vi "AMI_SetCampo.vi"(6 "error in (no error)":errorcluster, 7 "Index":i8) -> (0 "error out":errorcluster, 1 "resulting string Z":string="Set Magnetic Field 1000.000Tesla at 100.000Tesla/min, Linear, Persistent, Sweep&meas", 2 "resulting string Y":string="Set Magnetic Field 1000.000Tesla at 100.000Tesla/min, Linear, Persistent, Sweep&meas", 3 "resulting string X":string="Set Magnetic Field 1000.000Tesla at 100.000Tesla/min, Linear, Persistent, Sweep&meas")   [LabVIEW 2017]
doc: "Use this template to create a dialog box. This template polls the state of the buttons on the front panel and does not use events. Use the Dialog Using Events template (not available in Base package) to create a dialog box with event handling."
panel:
  out "Z Field Units":u16(ring)=1 items=["KGauss", "Tesla"]
  out "Z Ramp Units":u16(ring)=1 items=["Per SECOND", "Per MINUTE"]
  out "Y Field Units":u16(ring)=1 items=["KGauss", "Tesla"]
  out "Y Ramp Units":u16(ring)=1 items=["Per SECOND", "Per MINUTE"]
  in  "Z campo":dbl=0.1
  in  "Z rate":dbl=0.03
  in  "Y campo":dbl=0.1
  in  "Y rate":dbl=0.03
  in  "Modo Rampa":u16(ring)=1 items=["RAMP", "PAUSE", "MANUAL UP", "MANUAL DOWN", "ZERO"]
  out "X Ramp Units":u16(ring)=1 items=["Per SECOND", "Per MINUTE"]
  out "X Field Units":u16(ring)=1 items=["KGauss", "Tesla"]
  out "Wait stability":bool=TRUE
  in  "Field Mode":i32(ring) items=["Persistent", "Driven"]
  in  "Approach":i32(ring) items=["Linear", "NoOvershoot", "Oscillate"]
  in  "X rate":dbl=0.03
  in  "X campo":dbl=0.1
  out "Cancelled?":bool
  in  "Cancel":bool
  in  "OK":bool
  # "Junio 2022 V2.0  a-sslcdms"
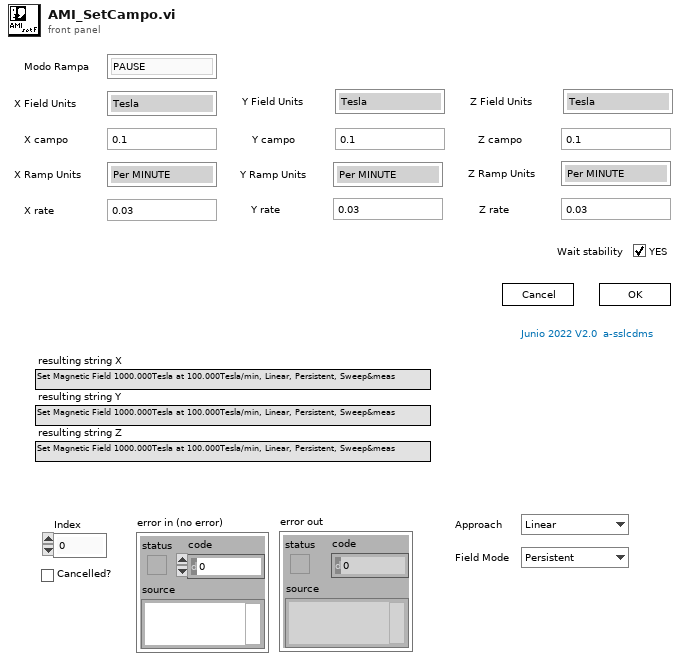
[diagram p1: front panel]
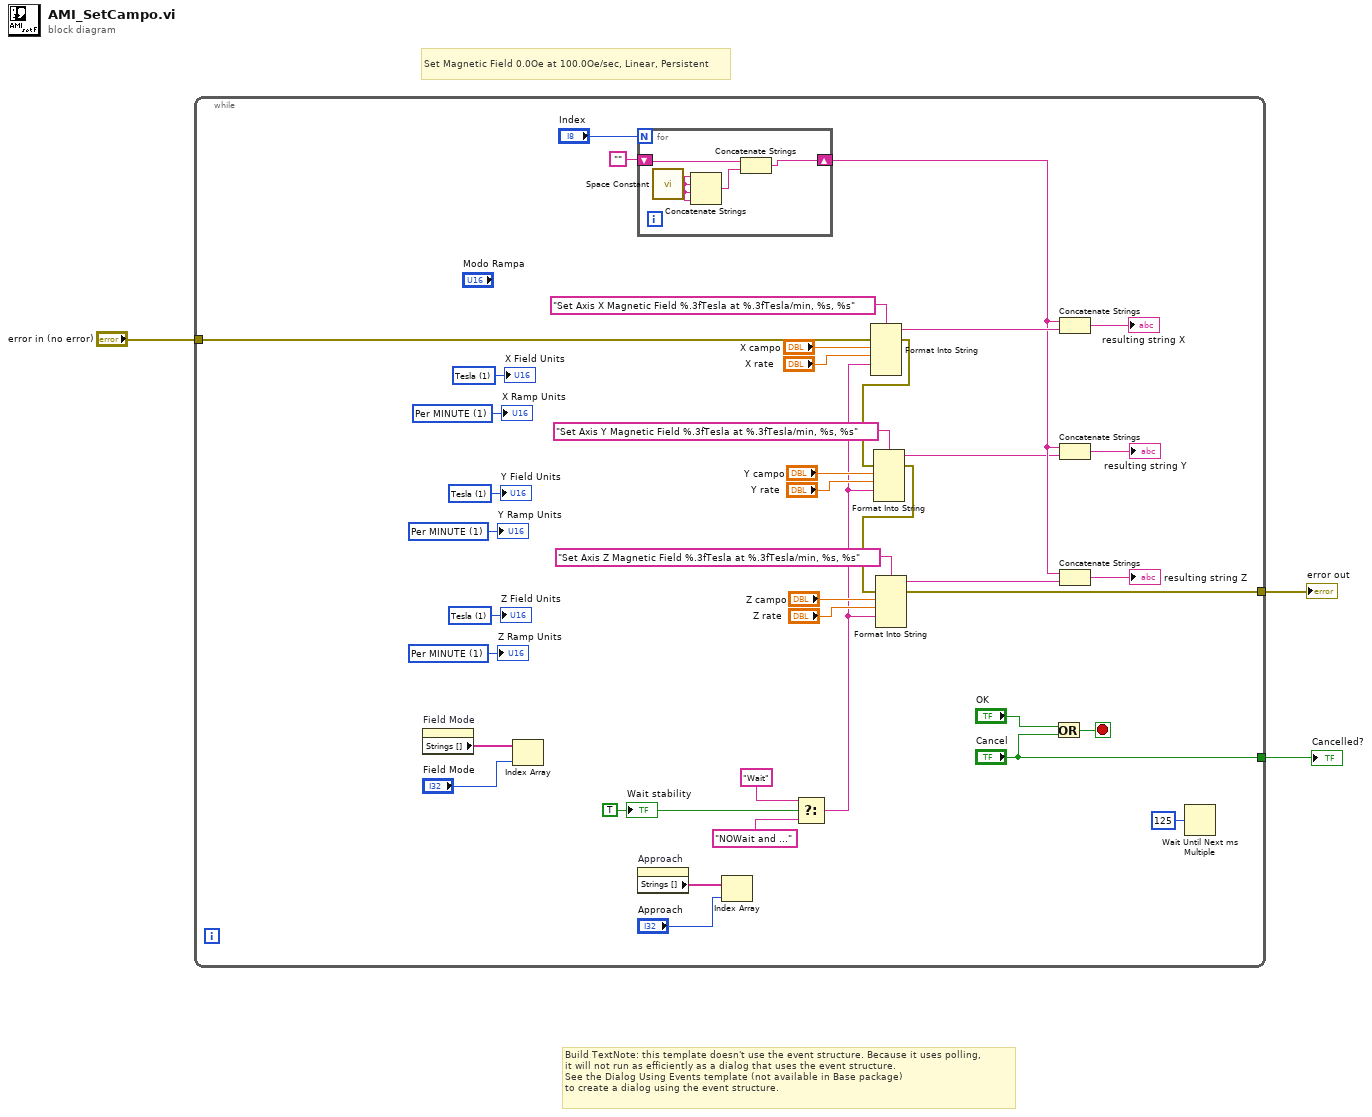
[diagram p0: block diagram]
diagram:
  # "Set Magnetic Field 0.0Oe at 100.0Oe/sec, Linear, Persistent"
  # "Build TextNote: this template doesn't use the event structure. Because it uses polling, \nit will not run as efficiently as a dialog that uses the event structure.\nSee the Dialog Using Events template (not available in Base package) \nto create a dialog using the event structure."
  n1 = while {
    tunnel: ["Cancel"] -> w3
    tunnel: [w9] -> w2
    tunnel: "error in (no error)" -> [w23]
    stop <- w42 stop-if-true
    w4 = u16 1 items=["Per SECOND", "Per MINUTE"] ("Ramp Units")
    w5 = u16 1 items=["KGauss", "Tesla"] ("Field Units")
    w7 = u16 1 items=["Per SECOND", "Per MINUTE"] ("Ramp Units")
    w6 = u16 1 items=["KGauss", "Tesla"] ("Field Units")
    w24 = u16 1 items=["Per SECOND", "Per MINUTE"] ("Ramp Units")
    w25 = u16 1 items=["KGauss", "Tesla"] ("Field Units")
    w28 = TRUE ("Wait stability")
    n2 = property on="Field Mode" class="Ring (strict)"() -> ("Strings []"=w31:string[])  [unwired: 2 in, 2 out]
    n3 = Index Array(array=w31, index="Field Mode") -> ()  [unwired: 1 out]
    n4 = for {
      N: "Index" -> [_]
      shift-right: [w46] -> w14
      shift-left: "" -> [w45]
      n5 = call <vilib>:"Space Constant.vi"() -> ("String"=w44:string)
      n6 = Concatenate Strings(w44, w44, w44, w44) -> (w47:string)
      n7 = Concatenate Strings(w45, w47) -> (w46:string)
    }
    n8 = property on="Approach" class="Ring (strict)"() -> ("Strings []"=w34:string[])  [unwired: 2 in, 2 out]
    n9 = Index Array(array=w34, index="Approach") -> ()  [unwired: 1 out]
    n10 = Select(t="Wait", s=w28, f="NOWait and ...") -> (s? t:f=w8:string)
    n11 = Format Into String(format string="Set Axis X Magnetic Field %.3fTesla at %.3fTesla/min, %s, %s", error in=w23, "X campo", "X rate", w8) -> (resulting string=w36:string, error out=w11:errorcluster)  [unwired: 2 in]
    n12 = Format Into String(format string="Set Axis Y Magnetic Field %.3fTesla at %.3fTesla/min, %s, %s", error in=w11, "Y campo", "Y rate", w8) -> (resulting string=w12:string, error out=w10:errorcluster)  [unwired: 2 in]
    n13 = Format Into String(format string="Set Axis Z Magnetic Field %.3fTesla at %.3fTesla/min, %s, %s", error in=w10, "Z campo", "Z rate", w8) -> (resulting string=w13:string, error out=w9:errorcluster)  [unwired: 2 in]
    n14 = Or(x="OK", y="Cancel") -> (x .or. y?=w42:bool)
    n15 = Concatenate Strings(w14, w36) -> (→"resulting string X":string)
    n16 = Concatenate Strings(w14, w12) -> (→"resulting string Y":string)
    n17 = Concatenate Strings(w14, w13) -> (→"resulting string Z":string)
    n18 = Wait Until Next ms Multiple(millisecond multiple=u32 125) -> ()  [unwired: 1 out]
    "Wait stability" <- w28
    "X Field Units" <- w25
    "X Ramp Units" <- w24
    "Y Field Units" <- w6
    "Y Ramp Units" <- w7
    "Z Field Units" <- w5
    "Z Ramp Units" <- w4
  }
  "Cancelled?" <- w3
  "error out" <- w2
